vi "HTTP_response_status.vi"(3 "error in (no error)":errorcluster, 4 "body":string, 5 "headers":string, 6 "HTTP status":string(combo)="201 CREATED") -> (0 "error out":errorcluster, 2 "Status":T1={"headers"="", "body"="", "ID"="", "Saved"=TRUE})   [LabVIEW 2013, in "Rinocloud Library.lvlib"]
uses:
  i3 JSON/JSON Parsing/Get Object Parameter Files/Get Object Parameter - Numeric.vi
  Rinocloud Library.lvlib
  i3 JSON/i3-json.lvlib
panel:
  out "offset of match":i32
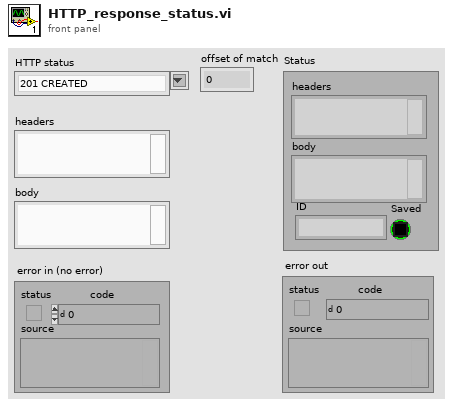
[diagram p1: front panel]
types:
  T1 = cluster{"headers":string, "body":string, "ID":string, "Saved":bool}
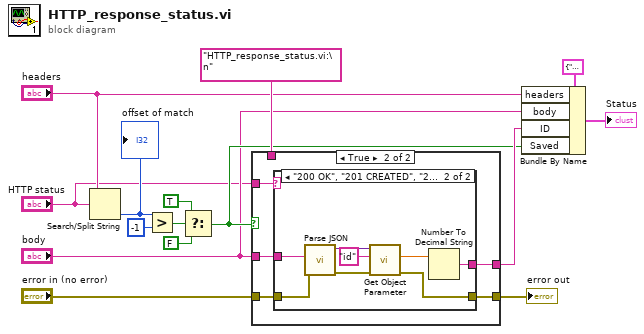
[diagram p0: block diagram]
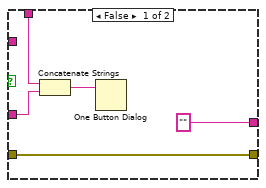
[diagram p2: hidden frame]
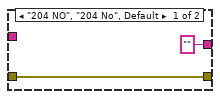
[diagram p3: hidden frame]
diagram:
  n1 = Search/Split String(string="headers", search string/char (-)="HTTP status") -> (offset of match=w15:i32)  [unwired: 1 in, 2 out]
  "offset of match" <- w15
  n2 = Greater?(x=w15, y=-1) -> (0:w13:bool)
  n3 = Select(t=TRUE, s=w13, f=FALSE) -> (s? t:f=w4:bool)
  n4 = case shown="True" w4 {
    tunnel: "body" -> [w18 w25]
    tunnel: ["" w22] -> w6
    tunnel: "error in (no error)" -> [w17 w24]
    tunnel: [w17 w23] -> w9
    tunnel: "HTTP_response_status.vi:\n" -> [w19 _]
    tunnel: "HTTP status" -> [_ w21]
    frame False {
      n5 = Concatenate Strings(w19, w18) -> (w16:string)
      n6 = One Button Dialog(message=w16) -> ()  [unwired: 1 in, 1 out]
    }
    frame True {
      n7 = case shown="\"200 OK\", \"201 CREATED\", \"201 Created\"" w21 {
        tunnel: w25 -> [_ w32]
        tunnel: w24 -> [w27 w31]
        tunnel: [w27 w30] -> w23
        tunnel: ["" w29] -> w22
        frame "204 NO", "204 No", Default {
        }
        frame "200 OK", "201 CREATED", "201 Created" {
          n8 = call "Parse JSON.vi"("error in (no error)"=w31, "JSON String"=w32) -> ("error out"=w35:errorcluster, "JSON Tree"=w33:variant)  [unwired: 6 in, 2 out]
          n9 = call-poly "Get Object Parameter.vi"("error in (no error)"=w35, "Parameter Name"="id", "JSON Tree In (JSON Object)"=w33) -> ("error out"=w30:errorcluster, "Double Value"=w28:dbl)  [unwired: 5 in, 2 out]
          n10 = Number To Decimal String(number=w28) -> (decimal integer string=w29:string)  [unwired: 1 in]
        }
      }
    }
  }
  "error out" <- w9
  n11 = Bundle By Name(cluster=T1 {"headers"="", "body"="", "ID"="", "Saved"=TRUE} ("Status 2"), "headers"="headers", "body"="body", "ID"=w6, "Saved"=w4) -> (→"Status":T1)
